vi "Kinesis - UDXC.vi"() -> ()   [LabVIEW 2013]
uses:
  C:/Users/zizhang/OneDrive - THORLABS Inc/Documents/4. SW Project/UDXC/LabVIEW/Thorlabs.MotionControl.Controls.dll
  4. SW Project/UDXC/LabVIEW/Thorlabs.MotionControl.Controls.dll
  C:/Users/zizhang/OneDrive - THORLABS Inc/Documents/4. SW Project/UDXC/LabVIEW/Thorlabs.MotionControl.Benchtop.PiezoCLI.dll
  4. SW Project/UDXC/LabVIEW/Thorlabs.MotionControl.Benchtop.PiezoCLI.dll
panel:
  in  "Set Reference Speed (nm/s)":u32=10000000
  out "Current Position (nm)":i32
  in  "Set Target Position (nm)":i32=1000000
  in  "SerialNumber":string="122000001"
  in  "BenchtopUDXCControl":refnum<k24>(container)
  # "Thorlabs Hardware: UDXC - Compact ORIC Ultrasonic Piezoelectric Drive Stage Controller \nhttps://www.thorlabs.com/thorproduct.cfm?partnumber=UDXC\n\nDescription: This VI will enable you to communicate with UDXC series to control ultrasonic piezo stages. The VI will first connect and initialize the device, home the stage and move the stage to a specified location.\n\nInstructions: \n1) Connect your device to your PC & power the device. ensuring your stage/actutator is connected prior to power the device. For full device setup, the device product manual can be found on our website.\n2) Enter the device serial number, reference speed and the target position below.\n3) Ensure the device move path is clear for homing.\n4) Click 'Run' in the LabVIEW Toolbar which will attempt a connection. And a home command will be sent.\n5) Await for device to be available, the stage will move to the target position."
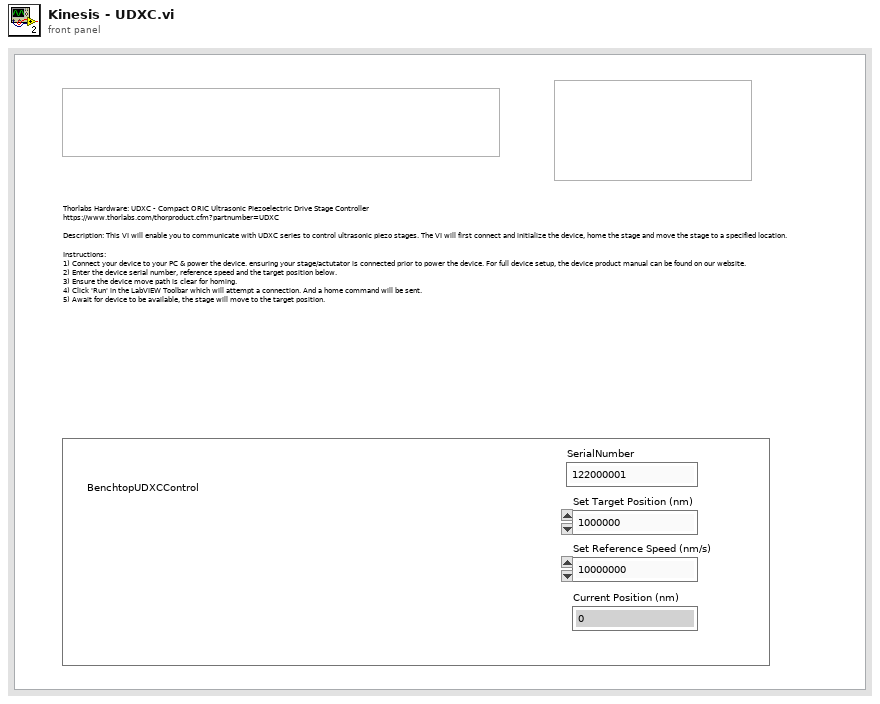
[diagram p1: front panel]
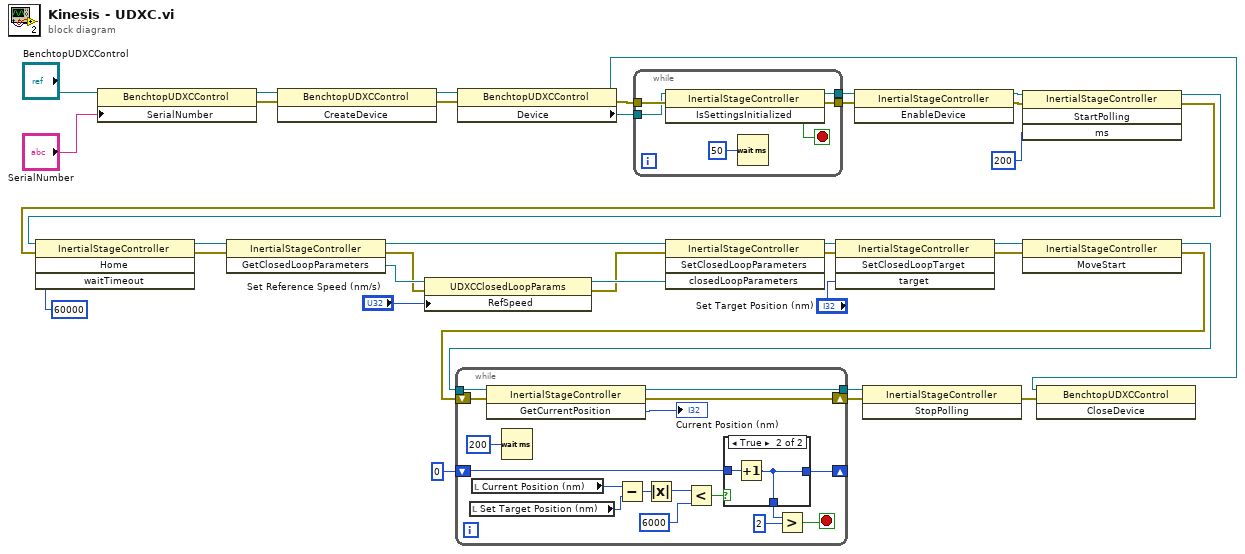
[diagram p0: block diagram]
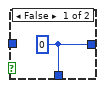
[diagram p2: hidden frame]
diagram:
  n1 = property class="BenchtopUDXCControl"(reference="BenchtopUDXCControl", "SerialNumber"="SerialNumber") -> (reference out=w34:refnum<k24>, error out=w33:errorcluster)  [unwired: 1 in]
  n2 = invoke class="BenchtopUDXCControl" method="CreateDevice"(reference=w34, error in=w33) -> (reference out=w32:refnum<k24>, error out=w31:errorcluster)  [unwired: 1 in, 1 out]
  n3 = property class="BenchtopUDXCControl"(reference=w32, error in=w31) -> (reference out=w29:refnum<k24>, error out=w30:errorcluster, "Device"=w21:refnum<k24>)
  n4 = while {
    tunnel: [w41] -> w28
    tunnel: w30 -> [w38]
    tunnel: [w39] -> w27
    tunnel: w21 -> [w37]
    stop <- w42 stop-if-true
    n5 = invoke class="InertialStageController" method="IsSettingsInitialized"(reference=w37, error in=w38) -> (reference out=w41:refnum<k24>, error out=w39:errorcluster, "IsSettingsInitialized"=w42:bool)  [unwired: 1 in]
    n6 = Wait (ms)(milliseconds to wait=u32 50) -> ()  [unwired: 1 out]
  }
  n7 = invoke class="InertialStageController" method="EnableDevice"(reference=w28, error in=w27) -> (reference out=w25:refnum<k24>, error out=w22:errorcluster)  [unwired: 1 in, 1 out]
  n8 = invoke class="InertialStageController" method="StartPolling"(reference=w25, error in=w22, "ms"=200) -> (reference out=w14:refnum<k24>, error out=w13:errorcluster)  [unwired: 1 in, 2 out]
  n9 = invoke class="InertialStageController" method="Home"(reference=w14, error in=w13, "waitTimeout"=60000) -> (reference out=w11:refnum<k24>, error out=w12:errorcluster)  [unwired: 1 in, 2 out]
  n10 = invoke class="InertialStageController" method="GetClosedLoopParameters"(reference=w11, error in=w12) -> (reference out=w10:refnum<k24>, error out=w4:errorcluster, "GetClosedLoopParameters"=w8:refnum<k24>)  [unwired: 1 in]
  n11 = property class="UDXCClosedLoopParams"(reference=w8, error in=w4, "RefSpeed"="Set Reference Speed (nm/s)") -> (reference out=w7:refnum<k24>, error out=w3:errorcluster)
  n12 = invoke class="InertialStageController" method="SetClosedLoopParameters"(reference=w10, error in=w3, "closedLoopParameters"=w7) -> (reference out=w1:refnum<k24>, error out=w9:errorcluster)  [unwired: 1 in, 2 out]
  n13 = invoke class="InertialStageController" method="SetClosedLoopTarget"(reference=w1, error in=w9, "target"="Set Target Position (nm)") -> (reference out=w19:refnum<k24>, error out=w18:errorcluster)  [unwired: 1 in, 2 out]
  n14 = invoke class="InertialStageController" method="MoveStart"(reference=w19, error in=w18) -> (reference out=w5:refnum<k24>, error out=w17:errorcluster)  [unwired: 1 in, 1 out]
  n15 = while {
    tunnel: [w56] -> w24
    shift-right: [w59] -> w23
    shift-left: w17 -> [w57]
    tunnel: w5 -> [w55]
    shift-right: [w44] -> _
    shift-left: 0 -> [w45]
    stop <- w46 stop-if-true
    n16 = local read "Set Target Position (nm)"() -> (w53:i32)
    n17 = local read "Current Position (nm)"() -> (w54:i32)
    n18 = invoke class="InertialStageController" method="GetCurrentPosition"(reference=w55, error in=w57) -> (reference out=w56:refnum<k24>, error out=w59:errorcluster, "GetCurrentPosition"=→"Current Position (nm)":i32)  [unwired: 1 in]
    n19 = Wait (ms)(milliseconds to wait=u32 200) -> ()  [unwired: 1 out]
    n20 = Subtract(x=w54, y=w53) -> (x-y=w52:i32)
    n21 = Absolute Value(x=w52) -> (abs(x)=w51:i32)
    n22 = Less?(x=w51, y=6000) -> (x < y?=w49:bool)
    n23 = case shown="True" w49 {
      tunnel: [w60 w61] -> w48
      tunnel: w45 -> [_ w62]
      tunnel: [w60 w61] -> w44
      frame False {
        w60 = 0
      }
      frame True {
        n24 = Increment(x=w62) -> (x+1=w61:i32)
      }
    }
    n25 = Greater?(x=w48, y=2) -> (0:w46:bool)
  }
  n26 = invoke class="InertialStageController" method="StopPolling"(reference=w24, error in=w23) -> (error out=w20:errorcluster)  [unwired: 1 in, 2 out]
  n27 = invoke class="BenchtopUDXCControl" method="CloseDevice"(reference=w29, error in=w20) -> ()  [unwired: 1 in, 3 out]
